vi "Generate trigger-Start of experiment.vi"(6 "Experiment start":bool, 8 "Acquiring":bool, 9 "start_ac_pulse":bool, 11 "Pulse width (ticks) -\"Start of Acq\" Trigger":u32=800000) -> (3 "\"Start of Acquisition\" trigger":bool)   [LabVIEW 2020]
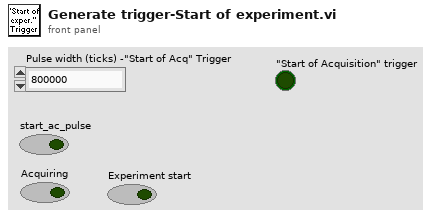
[diagram p1: front panel]
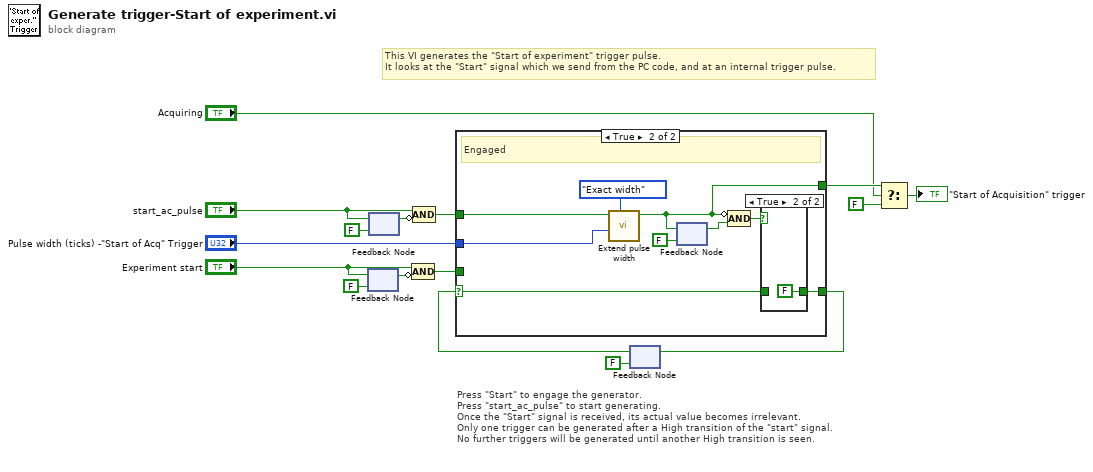
[diagram p0: block diagram]
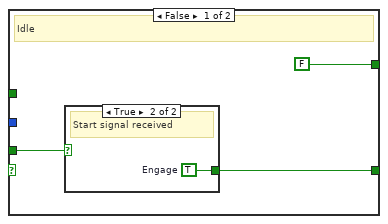
[diagram p2: hidden frame]
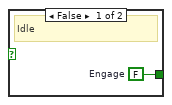
[diagram p3: hidden frame]
diagram:
  # "Press \"Start\" to engage the generator.\nPress \"start_ac_pulse\" to start generating.\nOnce the \"Start\" signal is received, its actual value becomes irrelevant.\nOnly one trigger can be generated after a High transition of the \"start\" signal.\nNo further triggers will be generated until another High transition is seen."
  # "This VI generates the \"Start of experiment\" trigger pulse.\nIt looks at the \"Start\" signal which we send from the PC code, and at an internal trigger pulse."
  n1 = feedback #1(FALSE ("start")) -> (w8:bool)
  n2 = feedback-in #1("Experiment start") -> ()
  n3 = feedback #2(FALSE ("start_ac_pulse")) -> (w12:bool)
  n4 = feedback-in #2("start_ac_pulse") -> ()
  n5 = Compound Arithmetic op=AND("Experiment start", invert w8) -> (w9:bool)
  n6 = Compound Arithmetic op=AND("start_ac_pulse", invert w12) -> (w5:bool)
  n7 = feedback #3(FALSE ("\"Start of Acquisition\" trigger")) -> (w10:bool)
  n8 = case shown="True" w10 {
    selector: w10 -> [_ w26]
    tunnel: w9 -> [w19 _]
    tunnel: [w18 w27] -> w13
    tunnel: w5 -> [_ w25]
    tunnel: [FALSE ("\"Start of Acquisition\" trigger") w24] -> w3
    tunnel: "Pulse width (ticks) -\"Start of Acq\" Trigger" -> [_ w23]
    frame False {
      # "Idle"
      n9 = case shown="True" w19 {
        tunnel: [w20 w21] -> w18
        frame False {
          w20 = FALSE  # Engage
          # "Idle"
        }
        frame True {
          w21 = TRUE  # Engage
          # "Start signal received"
        }
      }
    }
    frame True {
      # "Engaged"
      n10 = call "Extend pulse width.vi"("Function"=enum16{"Minimum width", "Exact width"}."Exact width", "Pulse width (ticks)(80000=1ms @80MHz)"=w23, "Input signal"=w25) -> ("Output signal"=w24:bool)  [unwired: 8 in]
      n11 = feedback #4(FALSE ("start_ac_pulse")) -> (w29:bool)
      n12 = feedback-in #4(w24) -> ()
      n13 = Compound Arithmetic op=AND(invert w24, w29) -> (w28:bool)
      n14 = case shown="True" w28 {
        tunnel: [w31 FALSE ("\"Start of Acquisition\" trigger")] -> w27
        tunnel: w26 -> [w31 _]
        frame False {
        }
        frame True {
        }
      }
    }
  }
  n15 = feedback-in #3(w13) -> ()
  n16 = Select(t=w3, s="Acquiring", f=FALSE) -> (s? t:f=→"\"Start of Acquisition\" trigger":bool)
